vi "Scan for Active Sessions - Observer.vi"() -> ()   [LabVIEW 2025]
uses:
  CLI Configurator/NetworkObjects Command.ctl
panel:
  out "Connections":map{string, string}(c390)
  in  "Clear":bool
  in  "Scan Timeout, ms":i32=50
  out "Current Scanning IP":string
  in  "Scan All Subnet Always":bool=TRUE
  in  "Stop Scanning":bool
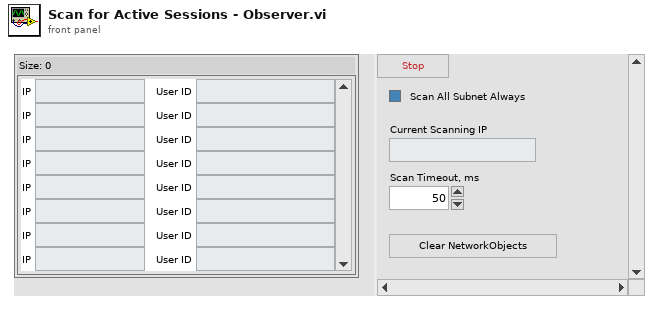
[diagram p1: front panel]
types:
  T1 = typedef "NetworkObjects Command.ctl" = enum16{"add computer", "add location", "clear", "dump", "export", "import", "list", "remove"}
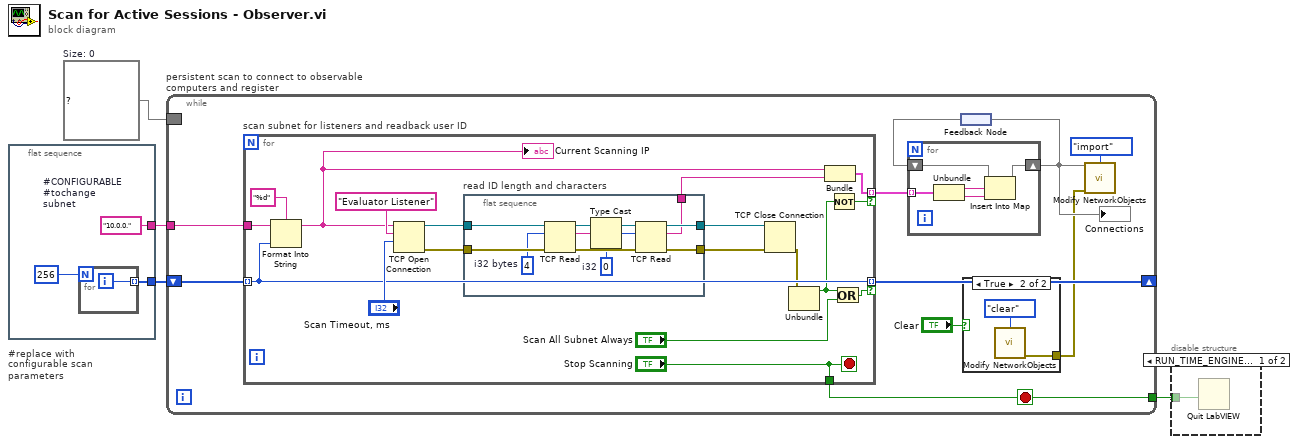
[diagram p0: block diagram]
diagram:
  w3 = map{string, string} {}  # Size: 0
  n1 = flat-sequence "#replace with configurable scan parameters" {
    tunnel: [w6] -> w4
    tunnel: [w5] -> w1
    frame #0 {
      w5 = "10.0.0."  # #CONFIGURABLE #tochange subnet
      n2 = for {
        N: 256 -> [_]
        tunnel: [w8] -> w6 mode=indexing
        i -> [w8]
      }
    }
  }
  n3 = while "persistent scan to connect to observable computers and register" {
    shift-right: [w17] -> _
    shift-left: w4 -> [w18]
    border: w3 -> [_]
    tunnel: [w14] -> w2
    tunnel: w1 -> [w13]
    stop <- w14 stop-if-true
    n4 = for "scan subnet for listeners and readback user ID" {
      tunnel: w18 -> [w41] mode=indexing
      tunnel: [w41] -> w17 mode=indexing if=w33
      tunnel: ["Stop Scanning"] -> w14
      tunnel: [w35] -> w16 mode=indexing if=w38
      tunnel: w13 -> [w26]
      stop <- "Stop Scanning" stop-if-true
      n5 = Format Into String(format string="%d", initial string=w26, w41) -> (resulting string=w31:string)  [unwired: 1 in, 1 out]
      "Current Scanning IP" <- w31
      n6 = TCP Open Connection(address=w31, remote port or service name="Evaluator Listener" ("format string"), timeout ms (60000)="Scan Timeout, ms") -> (connection ID=w37:refnum<k5>, error out=w36:errorcluster)  [unwired: 2 in]
      n7 = flat-sequence "read ID length and characters" {
        tunnel: w37 -> [w54]
        tunnel: w36 -> [w51]
        tunnel: [w47] -> w30
        tunnel: [w46] -> w28
        tunnel: [w45] -> w27
        frame #0 {
          w50 = 0  # i32
          w44 = 4  # i32 bytes
          n8 = TCP Read(connection ID=w54, bytes to read=w44, error in (no error)=w51) -> (connection ID out=w53:refnum<k5>, data out=w49:string, error out=w52:errorcluster)  [unwired: 2 in]
          n9 = Type Cast(type=w50, x=w49) -> (*(type *) &x=w48:i32)
          n10 = TCP Read(connection ID=w53, bytes to read=w48, error in (no error)=w52) -> (connection ID out=w46:refnum<k5>, data out=w45:string, error out=w47:errorcluster)  [unwired: 2 in]
        }
      }
      n11 = TCP Close Connection(connection ID=w28, error in (no error)=w30) -> (error out=w29:errorcluster)  [unwired: 1 in, 1 out]
      n12 = Unbundle(w29) -> ("status"=w39:bool)  [unwired: 2 out]
      n13 = Bundle(w31, "data out"=w27) -> (w35:cluster{string, "data out":string})  [unwired: 1 in]
      n14 = Not(x=w39) -> (.not. x?=w38:bool)
      n15 = Or(x=w39, y="Scan All Subnet Always") -> (x .or. y?=w33:bool)
    }
    n16 = feedback #1() -> (w15:map{string, string})
    n17 = for {
      tunnel: w16 -> [w25] mode=indexing
      shift-right: [w21] -> w12
      shift-left: w15 -> [w22]
      n18 = Unbundle(w25) -> (w24:string, "data out"=w23:string)
      n19 = Insert Into Map(map in=w22, key=w24, value=w23) -> (map out=w21:map{string, string})  [unwired: 2 out]
    }
    "Connections" <- w12
    n20 = feedback-in #1(w12) -> ()
    n21 = case shown="True" "Clear" {
      tunnel: [_ w19] -> w10
      frame False {
      }
      frame True {
        n22 = call "Modify NetworkObjects.vi"("Command (list)"=NetworkObjects_Command."clear") -> ("error out"=w19:errorcluster)  [unwired: 14 in]
      }
    }
    n23 = call "Modify NetworkObjects.vi"("Connections"=w12, "Command (list)"=NetworkObjects_Command."import", "error in"=w10) -> ()  [unwired: 12 in, 1 out]
  }
  n24 = disable-structure shown="RUN_TIME_ENGINE==True" {
    disable-tunnel: w2 -> [w55 _]
    frame condition #0 {
      n25 = Quit LabVIEW(quit? (T)=w55) -> ()
    }
    frame condition #1 (active) {
    }
  }
